vi "Loop_PDP_SEN.vi"() -> ()   [LabVIEW 2017, in "System_Status.lvlib"]
uses:
  System_Status.lvlib
  TypeDef Share All/CLUSTER_PDP_Status.ctl
  TypeDef Share All/CLUSTER_PDP_Faults.ctl
  Global Share All/Global_STOP.vi
  Global_SEN Write_Data.vi
panel:
  in  "PDP ID":i32
  out "Cycle Time (S)":dbl format="%.3g"
  in  "Target Time(ms)":u32=50
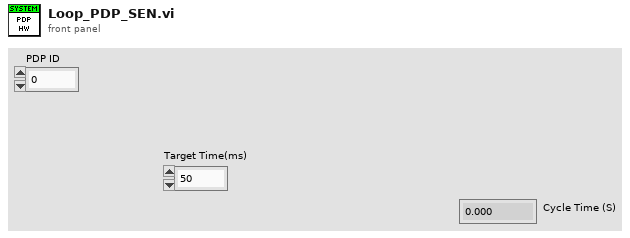
[diagram p1: front panel]
types:
  T1 = typedef "CLUSTER_PDP_Status.ctl" = cluster{"PDP Faults":T2, "All Currents (A)":dbl[], "Energy (J)":dbl, "Power (W)":dbl, "Voltage (V)":dbl}
  T2 = typedef "CLUSTER_PDP_Faults.ctl" = cluster{"Current Faults":bool[], "Batt V Fault":bool, "Temp Fault":bool, "HW Fault":bool}
  T3 = cluster{"PDP ID":i32, "Target Time(ms)":u32, "Current Time":timestamp, "Previous Time":timestamp, "Cycle Time (S)":dbl, "PDP Status":T1}
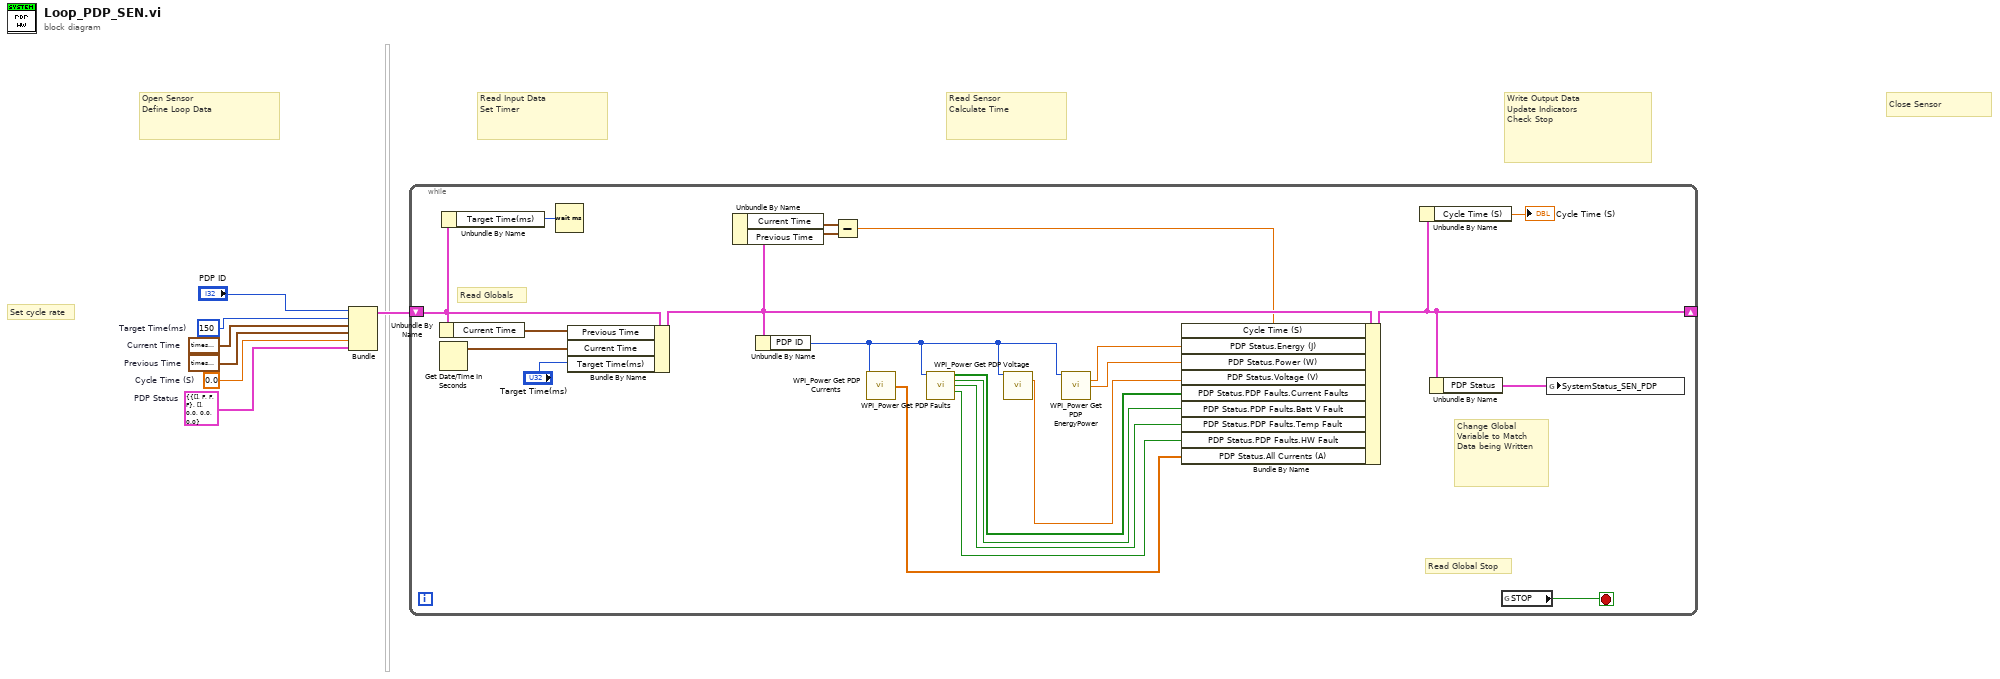
[diagram p0: block diagram]
diagram:
  w1 = T1 {"PDP Faults"={"Current Faults"=[], "Batt V Fault"=FALSE, "Temp Fault"=FALSE, "HW Fault"=FALSE}, "All Currents (A)"=[], "Energy (J)"=0.0, "Power (W)"=0.0, "Voltage (V)"=0.0}  # PDP Status
  w3 = 0.0  # Cycle Time (S)
  w7 = timestamp(0 s since 1904-01-01)  # Previous Time
  w6 = timestamp(0 s since 1904-01-01)  # Current Time
  w5 = u32 150  # Target Time(ms)
  # "Close Sensor"
  # "Write Output Data\nUpdate Indicators\nCheck Stop"
  # "Read Sensor\nCalculate Time"
  # "Read Input Data\nSet Timer"
  # "Open Sensor\nDefine Loop Data"
  # "Set cycle rate"
  n1 = Bundle("PDP ID"="PDP ID", "Target Time(ms)"=w5, "Current Time"=w6, "Previous Time"=w7, "Cycle Time (S)"=w3, "PDP Status"=w1) -> (w4:T3)  [unwired: 1 in]
  n2 = while {
    shift-right: [w19] -> _
    shift-left: w4 -> [w21]
    stop <- w29 stop-if-true
    # "Change Global\nVariable to Match\nData being Written"
    # "Read Globals"
    # "Read Global Stop"
    n3 = Unbundle By Name(w21) -> ("Current Time"=w26:timestamp)
    n4 = Get Date/Time In Seconds() -> (seconds since 1Jan1904=w27:timestamp)
    n5 = Unbundle By Name(w21) -> ("Target Time(ms)"=w20:u32)
    n6 = Wait (ms)(milliseconds to wait=w20) -> ()  [unwired: 1 out]
    n7 = Bundle By Name(cluster=w21, "Previous Time"=w26, "Current Time"=w27, "Target Time(ms)"="Target Time(ms)") -> (w22:T3)
    n8 = Unbundle By Name(w22) -> ("Current Time"=w25:timestamp, "Previous Time"=w24:timestamp)
    n9 = Unbundle By Name(w22) -> ("PDP ID"=w16:i32)
    n10 = Subtract(x=w25, y=w24) -> (x-y=w17:dbl)
    n11 = call <vilib>:"WPI_Power Get PDP Currents.vi"("Power Distribution Panel (0)"=w16) -> ("all currents (A)"=w15:dbl[])  [unwired: 12 in, 2 out]
    n12 = call <vilib>:"WPI_Power Get PDP Faults.vi"("Power Distribution Panel (0)"=w16) -> ("Current Faults"=w14:bool[], "Battery Voltage Fault"=w13:bool, "Temperature Fault"=w12:bool, "Hardware Fault"=w11:bool)  [unwired: 10 in, 1 out]
    n13 = call <vilib>:"WPI_Power Get PDP Voltage.vi"("Power Distribution Panel (0)"=w16) -> ("voltage (V)"=w10:dbl)  [unwired: 13 in, 1 out]
    n14 = call <vilib>:"WPI_Power Get PDP EnergyPower.vi"("Power Distribution Panel (0)"=w16) -> ("Energy (J)"=w8:dbl, "Power (W)"=w9:dbl)  [unwired: 12 in, 1 out]
    n15 = Bundle By Name(cluster=w22, "Cycle Time (S)"=w17, "PDP Status.Energy (J)"=w8, "PDP Status.Power (W)"=w9, "PDP Status.Voltage (V)"=w10, "PDP Status.PDP Faults.Current Faults"=w14, "PDP Status.PDP Faults.Batt V Fault"=w13, "PDP Status.PDP Faults.Temp Fault"=w12, "PDP Status.PDP Faults.HW Fault"=w11, "PDP Status.All Currents (A)"=w15) -> (w19:T3)
    n16 = Unbundle By Name(w19) -> ("Cycle Time (S)"=→"Cycle Time (S)":dbl)
    n17 = Unbundle By Name(w19) -> ("PDP Status"=w28:T1)
    n18 = global read "Global_STOP.vi" "STOP"() -> (w29:bool)
    n19 = global write "Global_SEN Write_Data.vi" "SystemStatus_SEN_PDP"(w28) -> ()
  }
